vi "Visible_by UT.vi"(9 "String":string) -> (0 "st1":bool, 1 "chREc":bool, 2 "Termp34":bool, 3 "Termp2":bool, 4 "UnitType":u16)   [LabVIEW 2017]
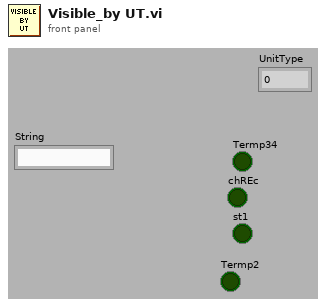
[diagram p1: front panel]
types:
  T1 = enum16{"Fuse25A", "PowerRider", "PowerRiderWE", "Hatal", "Palsan"}
  T2 = enum16{"Fuse25A", "PowerRider", "PowerRiderWE", "Hatal", "Palsan", "None", "PowerRider 12"}
  T3 = enum16{"Fuse25A", "PowerRider", "PowerRiderWE", "Hatal", "Plasan"}
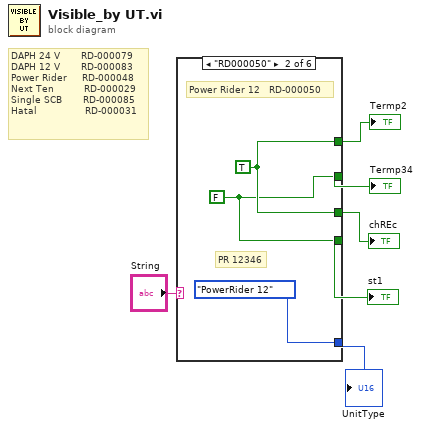
[diagram p0: block diagram]
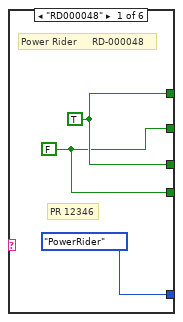
[diagram p2: hidden frame]
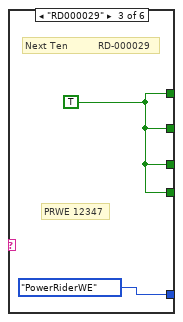
[diagram p3: hidden frame]
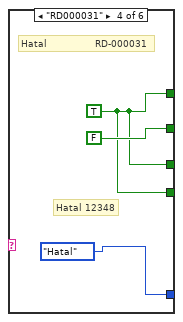
[diagram p4: hidden frame]
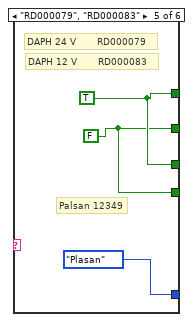
[diagram p5: hidden frame]
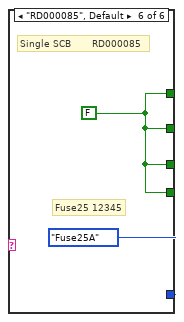
[diagram p6: hidden frame]
diagram:
  # "DAPH 24 V  \t    RD-000079\nDAPH 12 V  \t    RD-000083\nPower Rider \t   RD-000048\nNext Ten  \t       RD-000029\nSingle SCB       RD-000085 \nHatal                RD-000031"
  n1 = case shown="\"RD000050\"" "String" {
    tunnel: [T1."PowerRider" ("UnitType") T2."PowerRider 12" ("UnitType") T3."PowerRiderWE" ("UnitType") T3."Hatal" ("UnitType") T3."Plasan" ("UnitType") enum16{"Fuse25A", "PowerRider"}."Fuse25A" ("UnitType")] -> w5
    tunnel: [w8 w11 w13 w15 w19 w21] -> w2
    tunnel: [w7 w10 w13 FALSE w18 w21] -> w3
    tunnel: [w8 w11 w13 w15 w19 w21] -> w4
    tunnel: [w7 w10 w13 w15 w18 w21] -> w1
    frame "RD000048" {
      w8 = TRUE
      w7 = FALSE
      # "Power Rider \t   RD-000048"
      # "PR 12346"
    }
    frame "RD000050" {
      w11 = TRUE
      w10 = FALSE
      # "Power Rider 12   RD-000050"
      # "PR 12346"
    }
    frame "RD000029" {
      w13 = TRUE
      # "Next Ten  \t       RD-000029"
      # "PRWE 12347"
    }
    frame "RD000031" {
      w15 = TRUE
      # "Hatal                RD-000031"
      # "Hatal 12348"
    }
    frame "RD000079", "RD000083" {
      w18 = FALSE
      w19 = TRUE
      # "DAPH 12 V  \t    RD000083"
      # "DAPH 24 V  \t    RD000079"
      # "Palsan 12349"
    }
    frame "RD000085", Default {
      w21 = FALSE
      # "Single SCB       RD000085"
      # "Fuse25 12345"
    }
  }
  "UnitType" <- w5
  "Termp34" <- w3
  "Termp2" <- w4
  "chREc" <- w2
  "st1" <- w1
